vi "Read Scaled Data.vi"(8 "error in (no error)":errorcluster, 11 "1553 Component in":refnum<class "1553 Component.lvclass">) -> (0 "error out":errorcluster, 1 "Scaled Data":dbl[](array[numeric]), 2 "Parameters":string[](array[string]), 3 "1553 Component out":refnum<class "1553 Component.lvclass">)   [LabVIEW 2020, in "BCI-1553 API.lvlib" / "1553 Component.lvclass"]
doc: "Reads the parameters and values associated with this channel. Data will rescaled based on the scaling configuration of the parameter."
uses:
  1553 Component.lvclass
  1553 Component.lvclass/1553 Component.ctl
  1553 SubComponent/1553 SubComponent.lvclass
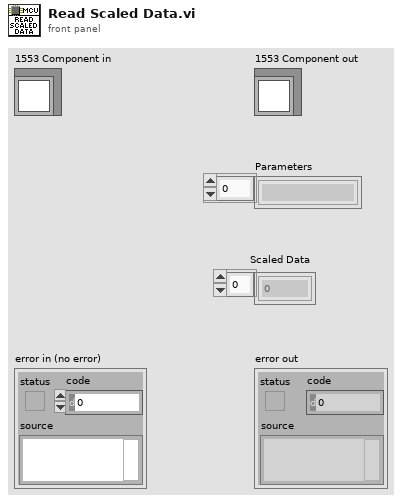
[diagram p1: front panel]
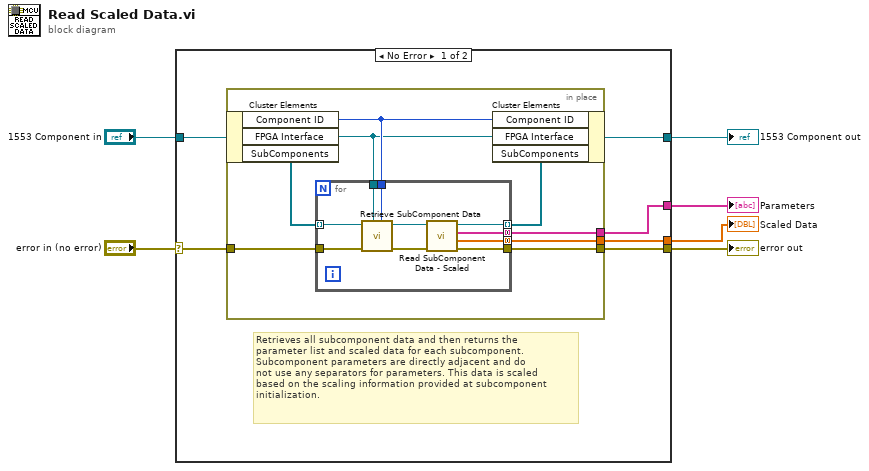
[diagram p0: block diagram]
diagram:
  n1 = case shown="No Error" "error in (no error)" {
    selector: "error in (no error)" -> [w11 w32]
    tunnel: [w10 w32] -> w5
    tunnel: [w9 w31] -> w4
    tunnel: "1553 Component in" -> [w12 w31]
    tunnel: [w8 _] -> w2
    tunnel: [w7 _] -> w1
    frame No Error {
      # "Retrieves all subcomponent data and then returns the\nparameter list and scaled data for each subcomponent.\nSubcomponent parameters are directly adjacent and do\nnot use any separators for parameters. This data is scaled\nbased on the scaling information provided at subcomponent\ninitialization."
      n2 = in-place {
        in-place-border: w11 -> [w16]
        in-place-border: [w15] -> w10
        in-place-border: [w14] -> w8
        in-place-border: [w13] -> w7
        n3 = in-place-cluster #1(w12) -> ("Component ID"=w20:u8, "FPGA Interface"=w17:refnum<class "FPGA Interface.lvclass">, "SubComponents"=w19:refnum<class "1553 SubComponent.lvclass">[])
        n4 = for {
          tunnel: w19 -> [w30] mode=indexing
          tunnel: [w25] -> w18 mode=indexing
          tunnel: w20 -> [w29]
          tunnel: w17 -> [w28]
          tunnel: w16 -> [w27]
          tunnel: [w23] -> w15
          tunnel: [w22] -> w14 mode=concatenating
          tunnel: [w21] -> w13 mode=concatenating
          n5 = call-dynamic "Retrieve SubComponent Data.vi"("Component ID"=w29, "FPGA Interface"=w28, "error in (no error)"=w27, "1553 SubComponent in"=w30) -> ("error out"=w24:errorcluster, "1553 SubComponent out"=w26:refnum<class "1553 SubComponent.lvclass">)  [unwired: 6 in]
          n6 = call-dynamic "Read SubComponent Data - Scaled.vi"("error in (no error)"=w24, "1553 SubComponent in"=w26) -> ("error out"=w23:errorcluster, "Scaled Data"=w22:dbl[], "Parameter"=w21:string[], "1553 SubComponent out"=w25:refnum<class "1553 SubComponent.lvclass">)  [unwired: 6 in]
        }
        n7 = in-place-cluster #1("Component ID"=w20, "FPGA Interface"=w17, "SubComponents"=w18) -> (w9:refnum<class "1553 Component.lvclass">)
      }
    }
    frame Error {
    }
  }
  "error out" <- w5
  "1553 Component out" <- w4
  "Scaled Data" <- w2
  "Parameters" <- w1
